vi "Clear.vi"(8 "Error Input":errorcluster, 10 "SessionId":string, 11 "LiteAgentSDK Input":refnum<k24>) -> (0 "Error Output":errorcluster, 3 "LiteAgentSDK Output":refnum<k24>)   [LabVIEW 2017, in "LiteAgentSDK.lvlib"]
uses:
  LiteAgentSDK.lvlib
  C:/Users/Jan/Projects/LiteAgentSDK-LabVIEW/Source/Bin/LiteAgentSDK.LabVIEW.dll
  Bin/LiteAgentSDK.LabVIEW.dll
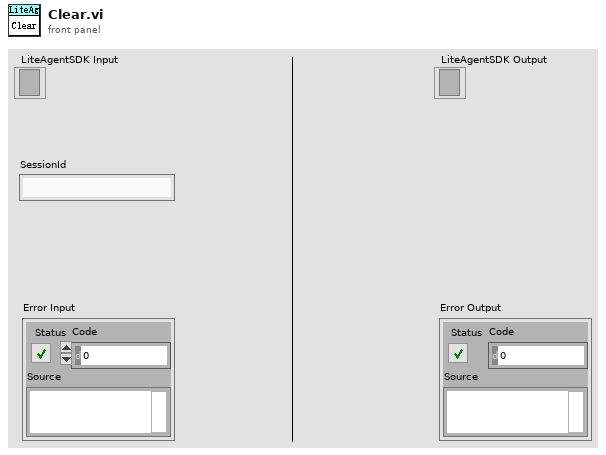
[diagram p1: front panel]
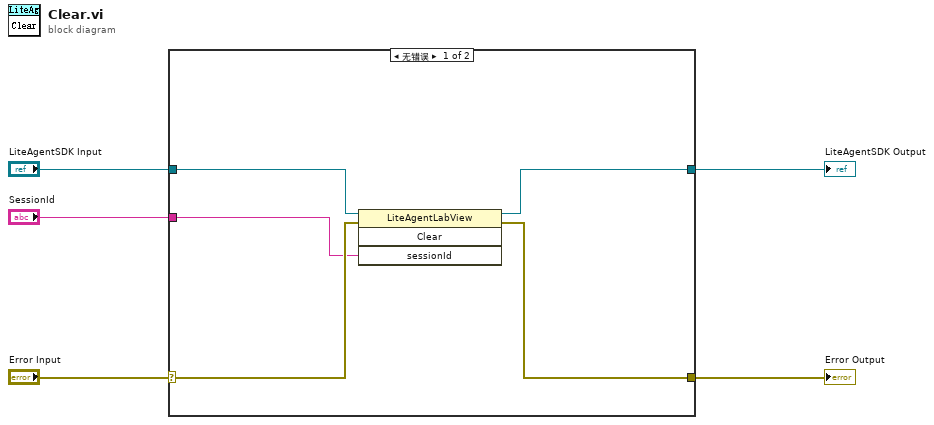
[diagram p0: block diagram]
diagram:
  n1 = case shown="无错误" "Error Input" {
    selector: "Error Input" -> [w10 w11]
    tunnel: "LiteAgentSDK Input" -> [w9 w12]
    tunnel: [w8 w12] -> w1
    tunnel: [w7 w11] -> w4
    tunnel: "SessionId" -> [w6 _]
    frame No Error {
      n2 = invoke on="调用节点" class="LiteAgentLabView" method="Clear"(reference=w9, error in=w10, "sessionId"=w6) -> (reference out=w8:refnum<k24>, error out=w7:errorcluster)  [unwired: 1 in, 2 out]
    }
    frame Error {
    }
  }
  "Error Output" <- w4
  "LiteAgentSDK Output" <- w1
